vi "报警信息.vi"(8 "error in (no error)":errorcluster, 10 "报警信息":string, 11 "设备":string) -> (0 "error out":errorcluster)   [LabVIEW 2016, in "斯坦道多参数.lvlib"]
uses:
  <vilib>/Utility/sysdir.llb/System Directory Type.ctl
  <vilib>/addons/database/Connection.llb/DB Tools Open Connec (String).vi
  <vilib>/addons/database/NI_Database_API.lvlib
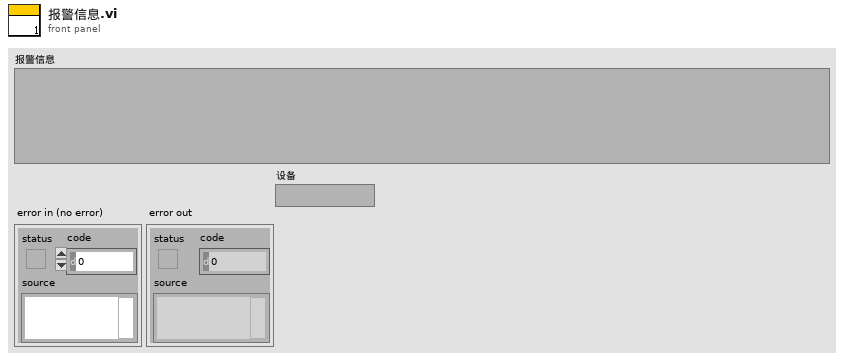
[diagram p1: front panel]
types:
  T1 = cluster{"时间标识":timestamp, "设备":string, "报警信息":string}
  T2 = typedef "System Directory Type.ctl" = i32
  T3 = typedef "NI_Database_API.lvlib/Conn ObjectReference.ctl" = refnum<k1>
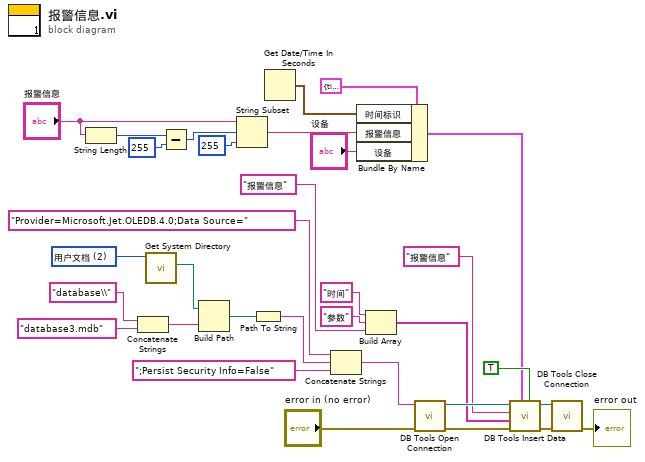
[diagram p0: block diagram]
diagram:
  w26 = T2 2 items=["用户目录"=0, "用户桌面"=1, "用户文档"=2, "用户应用程序数据"=3, "用户设置"=4, "用户临时目录"=5, "公共文档"=6, "公共应用程序数据"=7, "公共设置"=8, "公共缓存"=13, "系统核心库"=9, "系统安装库"=10, "应用程序文件"=11, "启动盘根目录"=12] ("system directory type")
  n1 = String Length(string="报警信息") -> (length=w5:i32)
  n2 = Concatenate Strings("database\\" ("condition"), "database3.mdb" ("database")) -> (w18:string)
  n3 = call <vilib>:"Get System Directory.vi"("system directory type"=w26) -> ("system directory"=w24:path)  [unwired: 10 in]
  n4 = Subtract(x=w5, y=255 ("长度（剩余）")) -> (x-y=w3:i32)
  n5 = Build Path(base path=w24, name or relative path=w18) -> (appended path=w23:path)
  n6 = String Subset(string="报警信息", offset (0)=w3, length (rest)=255 ("长度（剩余）")) -> (substring=w2:string)
  n7 = Path To String(path=w23) -> (string=w22:string)
  n8 = Get Date/Time In Seconds() -> (seconds since 1Jan1904=w11:timestamp)
  n9 = Concatenate Strings("Provider=Microsoft.Jet.OLEDB.4.0;Data Source=" ("condition"), w22, ";Persist Security Info=False" ("condition")) -> (w20:string)
  n10 = Bundle By Name(cluster=T1 {"时间标识"=timestamp(0 s since 1904-01-01), "设备"="多参数", "报警信息"=""} ("data in"), "时间标识"=w11, "报警信息"=w2, "设备"="设备") -> (w10:T1)
  n11 = Build Array("时间", "参数" ("元素"), "报警信息") -> (w14:string[])
  n12 = call-poly <vilib>:"DB Tools Open Connection.vi"("error in (no error)"="error in (no error)", "connection information"=w20) -> ("error out"=w16:errorcluster, "connection reference"=w17:T3)  [unwired: 6 in]
  n13 = call <vilib>:"DB Tools Insert Data.vi"("create table? (F)"=TRUE, "data"=w10, "error in (no error)"=w16, "columns"=w14, "table"="报警信息", "connection reference"=w17) -> ("error out"=w28:errorcluster, "connection reference out"=w29:T3)  [unwired: 4 in]
  n14 = call <vilib>:"DB Tools Close Connection.vi"("error in (no error)"=w28, "connection reference"=w29) -> ("error out"=→"error out":errorcluster)  [unwired: 5 in]
